vi "MergeRows.vi"(8 "error in (no error)":errorcluster, 9 "RowContent(Slave)":string[](array[string]), 10 "RowContent(Master)":string[](array[string]), 11 "ReportList":refnum<class "ReportList.lvclass">) -> (0 "error out":errorcluster, 2 "NewContents":string[](array[string]), 3 "ReportList Out":refnum<class "ReportList.lvclass">)   [LabVIEW 2015, in "ReportList.lvclass"]
uses:
  _reportList/ReportList.lvclass
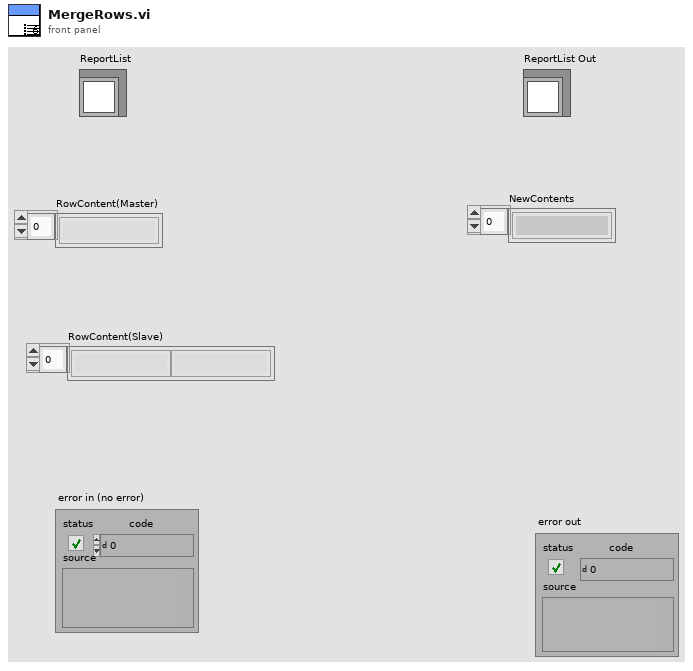
[diagram p1: front panel]
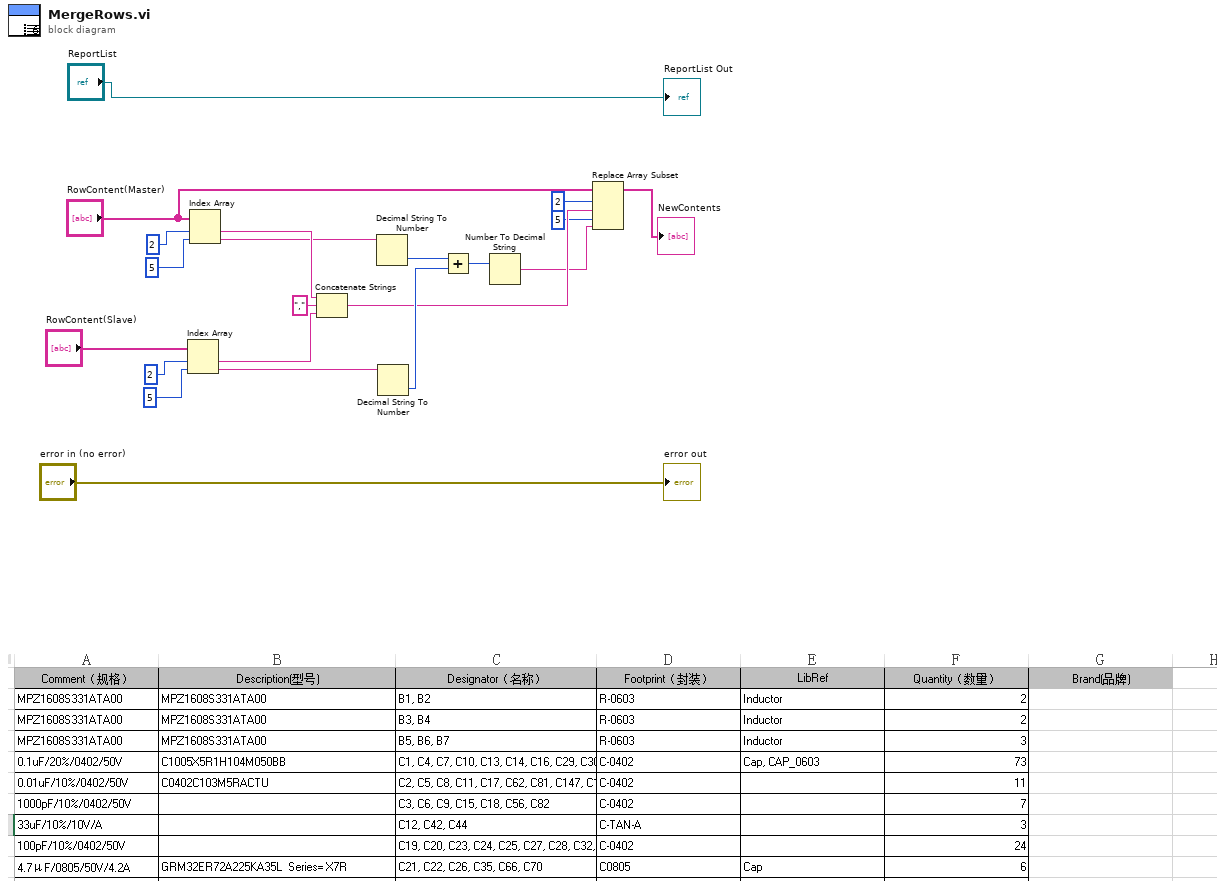
[diagram p0: block diagram]
diagram:
  n1 = Index Array(array="RowContent(Slave)", index #1=2 ("index"), index #2=5 ("index")) -> (element #1=w14:string, element #2=w12:string)
  n2 = Index Array(array="RowContent(Master)", index #1=2 ("index"), index #2=5 ("index")) -> (element #1=w16:string, element #2=w13:string)
  n3 = Concatenate Strings(w16, "," ("string"), w14) -> (w6:string)
  n4 = Decimal String To Number(string=w13) -> (number=w11:i32)  [unwired: 2 in, 1 out]
  n5 = Decimal String To Number(string=w12) -> (number=w10:i32)  [unwired: 2 in, 1 out]
  n6 = Add(x=w11, y=w10) -> (x+y=w8:i32)
  n7 = Number To Decimal String(number=w8) -> (decimal integer string=w4:string)  [unwired: 1 in]
  n8 = Replace Array Subset(array="RowContent(Master)", new element #1=w6, index #1=2 ("index"), new element #2=w4, index #2=5 ("index")) -> (→"NewContents":string[])
  "error out" <- "error in (no error)"
  "ReportList Out" <- "ReportList"
